vi "proc_resizeRescaleMemory.vi"(8 "to_height":i32, 9 "to_width":i32, 10 "Image Pixels (I16)":i16[][](array[numeric]), 11 "handle":i32) -> (0 "Image Pixels (I16) out":i16[][](array[numeric]), 3 "handle out":i32)   [LabVIEW 2010]
uses:
  lib/MWT.dll
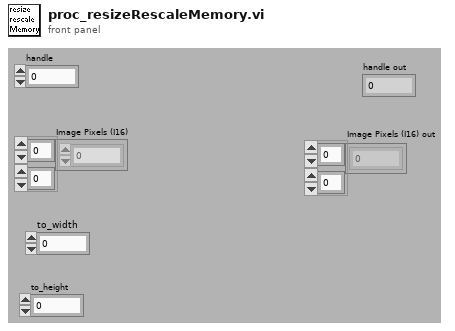
[diagram p1: front panel]
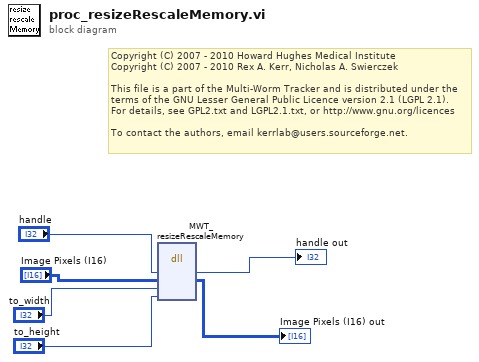
[diagram p0: block diagram]
diagram:
  # "Copyright (C) 2007 - 2010 Howard Hughes Medical Institute\nCopyright (C) 2007 - 2010 Rex A. Kerr, Nicholas A. Swierczek\n \nThis file is a part of the Multi-Worm Tracker and is distributed under the\nterms of the GNU Lesser General Public Licence version 2.1 (LGPL 2.1).\nFor details, see GPL2.txt and LGPL2.1.txt, or http://www.gnu.org/licences\n \nTo contact the authors, email kerrlab@users.sourceforge.net."
  n1 = dll-call lib="C:/MWT/lib/MWT.dll" fn="MWT_resizeRescaleMemory"("handle"="handle", "image_in"="Image Pixels (I16)", "width"="to_width", "height"="to_height") -> ("handle"=→"handle out":i32, "image_in"=→"Image Pixels (I16) out":i16[][])  [unwired: 6 in, 2 out]
